vi "testing template keys.vi"(6 "Test Station? (f)":bool, 8 "$$SEQLIST$$ (\"\")":string, 9 "$$SEQID$$ (\"\")":string, 10 "$$MODE$$ (\"\")":string, 11 "Keys In":T1) -> (3 "Keys Out":T1)   [LabVIEW 2011]
uses:
  Addons/internet/utils/keyedarr.llb/Keyed Array.ctl
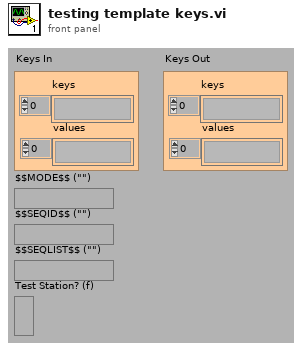
[diagram p1: front panel]
types:
  T1 = typedef "Keyed Array.ctl" = cluster{"keys":string[], "values":string[]}
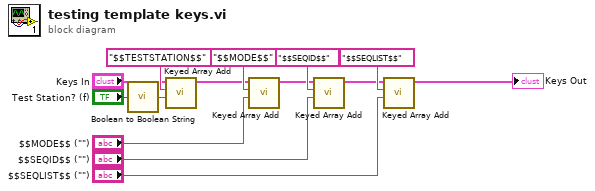
[diagram p0: block diagram]
diagram:
  n1 = call "Boolean to Boolean String.vi"("Boolean"="Test Station? (f)") -> ("Boolean string"=w7:string)  [unwired: 1 in]
  n2 = call "Keyed Array Add.vi"("value"=w7, "key"="$$TESTSTATION$$", "array in"="Keys In") -> ("array out"=w6:T1)  [unwired: 1 in, 3 out]
  n3 = call "Keyed Array Add.vi"("value"="$$MODE$$ (\"\")", "key"="$$MODE$$", "array in"=w6) -> ("array out"=w4:T1)  [unwired: 1 in, 3 out]
  n4 = call "Keyed Array Add.vi"("value"="$$SEQID$$ (\"\")", "key"="$$SEQID$$", "array in"=w4) -> ("array out"=w3:T1)  [unwired: 1 in, 3 out]
  n5 = call "Keyed Array Add.vi"("value"="$$SEQLIST$$ (\"\")", "key"="$$SEQLIST$$", "array in"=w3) -> ("array out"=→"Keys Out":T1)  [unwired: 1 in, 3 out]
